vi "Write signal from control.vi"(8 "Error In":errorcluster, 10 "Waveform Chart In":dynamicdata(graph), 11 "Display Panel.lvlib:Display Panel V3.lvclass In":refnum<class "Display Panel V3.lvclass">) -> (0 "Error Out":errorcluster, 3 "Ref Out":refnum<class "Display Panel V3.lvclass">)   [LabVIEW 2014, in "Display Panel.lvlib" / "Display Panel V3.lvclass"]
uses:
  Display Panel V3.lvclass
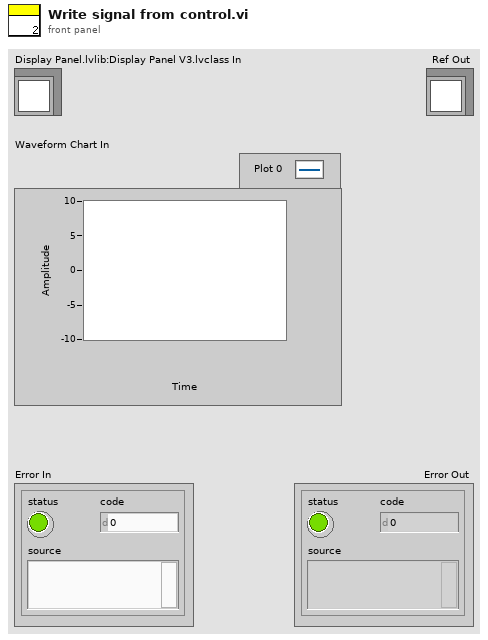
[diagram p1: front panel]
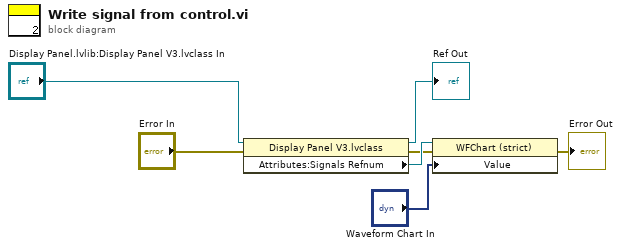
[diagram p0: block diagram]
diagram:
  n1 = property class="Display Panel V3.lvclass"(reference="Display Panel.lvlib:Display Panel V3.lvclass In", error in="Error In") -> (reference out=→"Ref Out":refnum<class "Display Panel V3.lvclass">, error out=w5:errorcluster, "Attributes:Signals Refnum"=w6:refnum<vi>)
  n2 = property class="WFChart (strict)"(reference=w6, error in=w5, "Value"="Waveform Chart In") -> (error out=→"Error Out":errorcluster)  [unwired: 1 out]
